vi "Configure Modulation.vi"   [LabVIEW 2012, in "Agilent 33XXX Series.lvlib"]
doc: "Configures the waveform modulation parameters."
uses:
  <instrlib>/Agilent 33XXX Series/Agilent 33XXX Series.lvlib
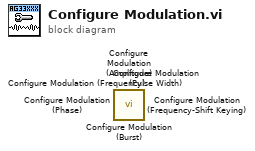
[diagram p0: block diagram]
diagram:
  n1 = call <instrlib>:"Configure Modulation (Burst).vi"() -> ()  [unwired: 14 in, 2 out]
  n2 = call <instrlib>:"Configure Modulation (Pulse Width).vi"() -> ()  [unwired: 14 in, 2 out]
  n3 = call <instrlib>:"Configure Modulation (Phase).vi"() -> ()  [unwired: 14 in, 2 out]
  n4 = call <instrlib>:"Configure Modulation (Frequency-Shift Keying).vi"() -> ()  [unwired: 14 in, 2 out]
  n5 = call <instrlib>:"Configure Modulation (Frequency).vi"() -> ()  [unwired: 14 in, 2 out]
  n6 = call <instrlib>:"Configure Modulation (Amplitude).vi"() -> ()  [unwired: 14 in, 2 out]
